vi "Is Point In Shape.vi"(8 "error in (no error)":errorcluster, 10 "Point":cluster{"Horizontal":i32, "Vertical":i32}, 11 "Line in":refnum<class "Line.lvclass">) -> (0 "error out":errorcluster, 2 "Point In Shape?":bool, 3 "Line out":refnum<class "Line.lvclass">)   [LabVIEW 2015, in "Line.lvclass"]
uses:
  Line.lvclass
  Interfaces/Shape/Shape.lvclass/Shape.ctl
  Interfaces/Shape/Shape.lvclass
  <vilib>/Analysis/NI_AALPro.lvlib
panel:
  # "NOTICE -- YOU MUST LEAVE THIS NOTICE IN PLACE.\n\nCopyright (c) 2017, LIANG LIU Shawn.Liu.cn@gmail.com\nAll rights reserved.\n\nRedistribution and use in source and binary forms, with or without modification, are permitted provided that the following conditions are met:\n-Redistributions of source code must retain the above copyright notice, this list of conditions and the following disclaimer.\n-Redistributions in binary form must reproduce the above copyright notice, this list of conditions and the following disclaimer in the documentation and/or other materials provided with the distribution.\n-Neither the name of the eLp nor the names of its contributors may be used to endorse or promote products derived from this software without specific prior written permission.\n\nTHIS SOFTWARE IS PROVIDED BY THE COPYRIGHT HOLDERS AND CONTRIBUTORS \"AS IS\" AND ANY EXPRESS OR IMPLIED WARRANTIES, INCLUDING, BUT NOT LIMITED TO, THE IMPLIED WARRANTIES OF MERCHANTABILITY AND FITNESS FOR A PARTICULAR PURPOSE ARE DISCLAIMED. IN NO EVENT SHALL THE COPYRIGHT HOLDER OR CONTRIBUTORS BE LIABLE FOR ANY DIRECT, INDIRECT, INCIDENTAL, SPECIAL, EXEMPLARY, OR CONSEQUENTIAL DAMAGES (INCLUDING, BUT NOT LIMITED TO, PROCUREMENT OF SUBSTITUTE GOODS OR SERVICES; LOSS OF USE, DATA, OR PROFITS; OR BUSINESS INTERRUPTION) HOWEVER CAUSED AND ON ANY THEORY OF LIABILITY, WHETHER IN CONTRACT, STRICT LIABILITY, OR TORT (INCLUDING NEGLIGENCE OR OTHERWISE) ARISING IN ANY WAY OUT OF THE USE OF THIS SOFTWARE, EVEN IF ADVISED OF THE POSSIBILITY OF SUCH DAMAGE."
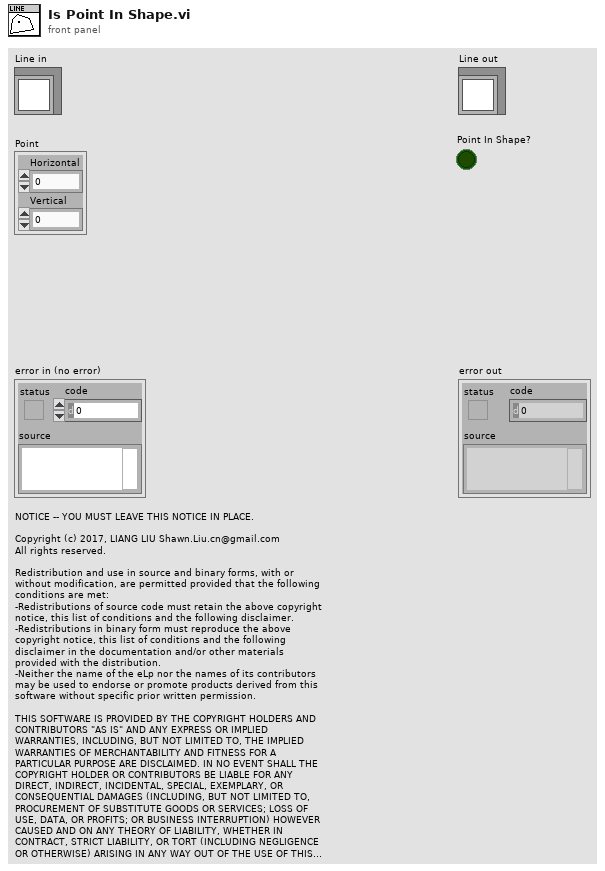
[diagram p1: front panel]
types:
  T1 = cluster{"left":i16, "top":i16, "right":i16, "bottom":i16}
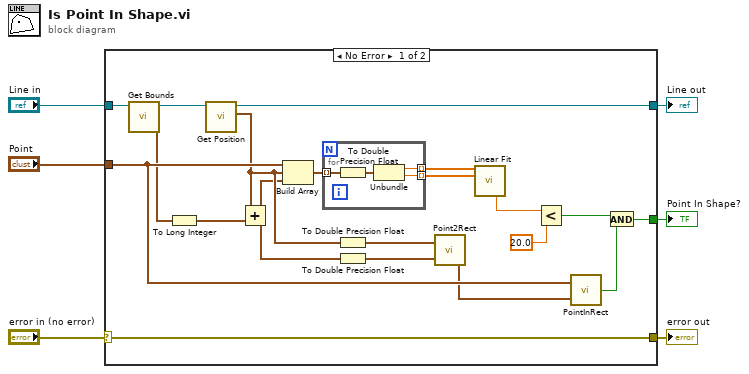
[diagram p0: block diagram]
diagram:
  n1 = case shown="No Error" "error in (no error)" {
    selector: "error in (no error)" -> [w22 w32]
    tunnel: "Line in" -> [w26 w31]
    tunnel: [w25 w31] -> w5
    tunnel: "Point" -> [w24 _]
    tunnel: [w23 _] -> w3
    tunnel: [w22 w32] -> w1
    frame No Error {
      n2 = call "Get Bounds.vi"("Shape in"=w26) -> ("Bounds"=w20:cluster{"Width":u32, "Height":u32}, "Shape out"=w21:refnum<class "Line.lvclass">)  [unwired: 9 in]
      n3 = To Long Integer(number=w20) -> (32bit integer=w10:cluster{"Width":i32, "Height":i32})
      n4 = call "Get Position.vi"("Shape in"=w21) -> ("Position"=w16:cluster{"Left":i32, "Top":i32}, "Shape out"=w25:refnum<class "Line.lvclass">)  [unwired: 9 in]
      n5 = Add(x=w16, y=w10) -> (x+y=w15:cluster{i32, i32})
      n6 = Build Array(w24, w16, w15) -> (w19:cluster{"Left":i32, "Top":i32}[])
      n7 = for {
        tunnel: w19 -> [w30] mode=indexing
        tunnel: [w29] -> w18 mode=indexing
        tunnel: [w27] -> w17 mode=indexing
        n8 = To Double Precision Float(number=w30) -> (double precision float=w28:cluster{"Left":dbl, "Top":dbl})
        n9 = Unbundle(w28) -> ("Left"=w29:dbl, "Top"=w27:dbl)
      }
      n10 = To Double Precision Float(number=w16) -> (double precision float=w9:cluster{"Left":dbl, "Top":dbl})
      n11 = To Double Precision Float(number=w15) -> (double precision float=w8:cluster{dbl, dbl})
      n12 = call <vilib>:"Point2Rect.vi"("point b"=w8, "point a"=w9) -> ("rect"=w14:T1)
      n13 = call <vilib>:"Linear Fit.vi"("Y"=w18, "X"=w17) -> ("residue"=w7:dbl)  [unwired: 9 in, 4 out]
      n14 = Less?(x=w7, y=20.0) -> (x < y?=w12:bool)
      n15 = call <vilib>:"PointInRect.vi"("rect"=w14, "point"=w24) -> ("pt in rect"=w11:bool)
      n16 = And(x=w12, y=w11) -> (x .and. y?=w23:bool)
    }
    frame Error {
    }
  }
  "error out" <- w1
  "Line out" <- w5
  "Point In Shape?" <- w3
